vi "add points.vi"(10 "Spacing":dbl=1.0, 11 "Waypoints":dbl[][](array[numeric])) -> (3 "Path":dbl[][](array[numeric]) format="%#.3f")   [LabVIEW 2018]
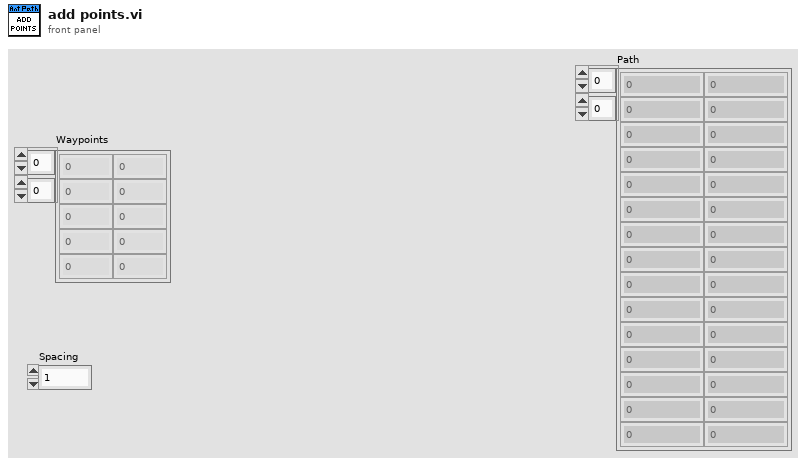
[diagram p1: front panel]
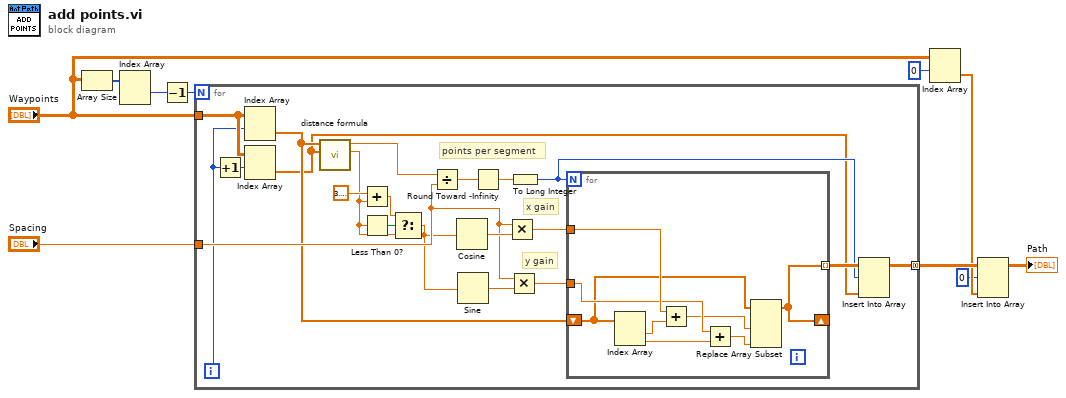
[diagram p0: block diagram]
diagram:
  n1 = Array Size(array="Waypoints") -> (size(s)=w10:i32[])
  n2 = Index Array(array=w10) -> (element #1=w9:i32)  [unwired: 2 in, 1 out]
  n3 = Decrement(x=w9) -> (x-1=w6:i32)
  n4 = for {
    N: w6 -> [_]
    tunnel: "Waypoints" -> [w30]
    tunnel: "Spacing" -> [w25]
    tunnel: [w20] -> w7 mode=concatenating
    i -> [w21]
    # "y gain"
    # "x gain"
    # "points per segment"
    n5 = Increment(x=w21) -> (x+1=w31:i32)
    n6 = Index Array(array=w30, index (row)=w21) -> (element=w22:dbl[])  [unwired: 1 in]
    n7 = Index Array(array=w30, index (row)=w31) -> (element=w16:dbl[])  [unwired: 1 in]
    n8 = call "distance formula.vi"("Point Y"=w16, "Point X"=w22) -> ("Angle (rad)"=w13:dbl, "Distance"=w18:dbl)  [unwired: 8 in]
    n9 = Add(x=3.141592653589793, y=w13) -> (x+y=w11:dbl)
    n10 = Less Than 0?(x=w13) -> (x < 0?=w14:bool)
    n11 = Select(t=w11, s=w14, f=w13) -> (s? t:f=w12:dbl)
    n12 = Divide(x=w18, y=w25) -> (x/y=w29:dbl)
    n13 = Cosine(x=w12) -> (cos(x)=w27:dbl)
    n14 = Sine(x=w12) -> (sin(x)=w26:dbl)
    n15 = Round Toward -Infinity(1:w29) -> (0:w28:dbl)
    n16 = Multiply(x=w25, y=w27) -> (x*y=w17:dbl)
    n17 = Multiply(x=w25, y=w26) -> (x*y=w24:dbl)
    n18 = To Long Integer(number=w28) -> (32bit integer=w19:i32)
    n19 = for {
      N: w19 -> [_]
      shift-right: [w32] -> _
      shift-left: w22 -> [w35]
      tunnel: w17 -> [w38]
      tunnel: w24 -> [w36]
      tunnel: [w32] -> w23 mode=indexing
      n20 = Index Array(array=w35) -> (element #1=w39:dbl, element #2=w37:dbl)  [unwired: 2 in]
      n21 = Add(x=w38, y=w39) -> (x+y=w34:dbl)
      n22 = Add(x=w36, y=w37) -> (x+y=w33:dbl)
      n23 = Replace Array Subset(array=w35, new element #1=w34, new element #2=w33) -> (w32:dbl[])  [unwired: 2 in]
    }
    n24 = Insert Into Array(array=w23, index (row)=w19, new element=w16) -> (w20:dbl[][])  [unwired: 1 in]
  }
  n25 = Index Array(array="Waypoints", index (row)=0) -> (element=w2:dbl[])  [unwired: 1 in]
  n26 = Insert Into Array(array=w7, index (row)=0, new element=w2) -> (→"Path":dbl[][])  [unwired: 1 in]
